vi "Get Cursor Values from Data.vi"(5 "octave spectra":T5(array[cluster]) {"band power" format="%.2f"; "nominal frequencies [Hz]" format="%.2f"}, 7 "octave info":T6[](array[typedef]) {"engineering units" items=["custom..."=0, "V"=1, "A"=21, "C"=30, "pC"=31, "s"=32, "-"=29, "Pa"=2, "N"=20, "g"=3, "m/s^2"=4, "m/s"=5, "m"=6, "mm/s"=12, "mm"=13, "micron/s"=14, "micron"=15, "in/s^2"=7, "in/s"=8, "in"=9, "mil/s"=10, "mil"=11, "rad/s^2"=16, "rad/s"=17, "rad"=18, "deg/s^2"=26, "deg/s"=27, "deg"=28, "RPM"=22, "cycle/s^2"=23, "Hz"=24, "cycle"=25, "strain"=19]; "dB reference" format="%.2e"; "weighting filter" items=["Linear", "A-weighting", "B-weighting", "C-weighting", "ITU-R 468-4", "Dolby", "CCITT", "C-message", "Wb", "Wc", "Wd", "We", "Wf", "Wh", "Wj", "Wk", "Wm", "AES17 20 kHz lowpass", "AES17 40 kHz lowpass", "AES17 20 kHz highpass", "AES17 40 kHz highpass"]}, 10 "Refnums for FP Objects":T1, 11 "Display State In":T2={"Graph Visible Items"={"Plot Legend"=FALSE, "Scale Legend"=FALSE, "Graph Palette"=FALSE, "Cursor Legend"=FALSE, "X Scrollbar"=FALSE}, "View Table"=FALSE, "Table Visible Items"={"Vertical Scrollbar"=FALSE, "Horizontal Scrollbar"=FALSE, "Row Headers"=FALSE, "Column Headers"=FALSE, "Vertical Lines"=FALSE, "Horizontal Lines"=FALSE}, "Header Font"={"Font Name"="", "Size"=0, "Bold"=FALSE, "Italic"=FALSE, "Underline"=FALSE, "Strikeout"=FALSE, "Color"=0}, "Cell Font"={"Font Name"="", "Size"=0, "Bold"=FALSE, "Italic"=FALSE, "Underline"=FALSE, "Strikeout"=FALSE, "Color"=0}, "Description and Tip..."={"Description"="", "Tip"=""}, "Moveable Splitter Position"=0, "Measurement Cursor Configuration"={"XY"={"enable XY"=FALSE, "Position (X)"=[], "Type"=enum."Absolute", "Y reference"=0.0, "color"=0}, "band"={"enable band"=FALSE, "B1"=0.0, "B2"=0.0, "Fixed bandwidth (B2-B1)"=0.0, "B1 color"=0, "B2 color"=0}, "harmonic"={"enable harmonics"=FALSE, "X reference (1X)"=0.0, "Maximum"=0, "Subset"=enum."All", "1X color"=0, "MX color"=0}, "sideband"={"enable sideband"=FALSE, "X center (C)"=0.0, "Sidebands"=0, "X spacing (s)"=0.0, "Center color"=0, "Sideband color"=0}}, "Cursors"={"List"=[], "Tags"=[]}, "X Increment"=0.0, "X Scale"={"Label Visible"=FALSE, "Label Text"="", "Mapping Mode"=0, "Format String"=""}, "Y Scale"={"Label Visible"=FALSE, "Label Text"="", "Mapping Mode"=0, "Format String"=""}, "Colors"={"background"=16777215, "major grid"=8355711, "minor grid"=12632256, "font"=0}, "desired spectrum view"={"scaling"={"linear/dB"=enum."no change", "dB reference"=0.0, "power/magnitude"=enum."no change", "view"=enum."no change"}, "spectral density"=enum."no change"}, "Plot Color Wheel"=[3381759, 32768, 982784, 4375295, 13827953, 13457919, 16757522, 4343295, 16728758, 12095254], "Plots"=[], "registered user events"=variant, "Lock 1X to Peak"=FALSE} caption="State" {"Y Scale"."Mapping Mode" items=["Linear", "Logarithmic", "dB"]; "X Scale"."Mapping Mode" items=["Linear", "Logarithmic"]}) -> (2 "value table":string[][](array[string]), 3 "Display State Out":T2={"Graph Visible Items"={"Plot Legend"=FALSE, "Scale Legend"=FALSE, "Graph Palette"=FALSE, "Cursor Legend"=FALSE, "X Scrollbar"=FALSE}, "View Table"=FALSE, "Table Visible Items"={"Vertical Scrollbar"=FALSE, "Horizontal Scrollbar"=FALSE, "Row Headers"=FALSE, "Column Headers"=FALSE, "Vertical Lines"=FALSE, "Horizontal Lines"=FALSE}, "Header Font"={"Font Name"="", "Size"=0, "Bold"=FALSE, "Italic"=FALSE, "Underline"=FALSE, "Strikeout"=FALSE, "Color"=0}, "Cell Font"={"Font Name"="", "Size"=0, "Bold"=FALSE, "Italic"=FALSE, "Underline"=FALSE, "Strikeout"=FALSE, "Color"=0}, "Description and Tip..."={"Description"="", "Tip"=""}, "Moveable Splitter Position"=0, "Measurement Cursor Configuration"={"XY"={"enable XY"=FALSE, "Position (X)"=[], "Type"=enum."Absolute", "Y reference"=0.0, "color"=0}, "band"={"enable band"=FALSE, "B1"=0.0, "B2"=0.0, "Fixed bandwidth (B2-B1)"=0.0, "B1 color"=0, "B2 color"=0}, "harmonic"={"enable harmonics"=FALSE, "X reference (1X)"=0.0, "Maximum"=0, "Subset"=enum."All", "1X color"=0, "MX color"=0}, "sideband"={"enable sideband"=FALSE, "X center (C)"=0.0, "Sidebands"=0, "X spacing (s)"=0.0, "Center color"=0, "Sideband color"=0}}, "Cursors"={"List"=[], "Tags"=[]}, "X Increment"=0.0, "X Scale"={"Label Visible"=FALSE, "Label Text"="", "Mapping Mode"=0, "Format String"=""}, "Y Scale"={"Label Visible"=FALSE, "Label Text"="", "Mapping Mode"=0, "Format String"=""}, "Colors"={"background"=16777215, "major grid"=8355711, "minor grid"=12632256, "font"=0}, "desired spectrum view"={"scaling"={"linear/dB"=enum."no change", "dB reference"=0.0, "power/magnitude"=enum."no change", "view"=enum."no change"}, "spectral density"=enum."no change"}, "Plot Color Wheel"=[3381759, 32768, 982784, 4375295, 13827953, 13457919, 16757522, 4343295, 16728758, 12095254], "Plots"=[], "registered user events"=variant, "Lock 1X to Peak"=FALSE} caption="State" {"Y Scale"."Mapping Mode" items=["Linear", "Logarithmic", "dB"]; "X Scale"."Mapping Mode" items=["Linear", "Logarithmic"]}, 4 "measurement names":string[](array[string]), 6 "channels":string[](array[string]))   [LabVIEW 2017, in "Octave with Cursors.xctl"]
doc: "This VI extracts the spectral values at the cursor positions. Based on the spectral data, Row Headers, Column Headers, and Values are written to the table."
uses:
  <vilib>/addons/_XControls/Octave with Cursors/Octave with Cursors.xctl
  <vilib>/addons/_XControls/Octave with Cursors/Controls/State.ctl
  <vilib>/Utility/miscctls.llb/LVFontTypeDef.ctl
  <vilib>/addons/_XControls/Octave with Cursors/Controls/Measurement Cursor Configuration.ctl
  <vilib>/addons/_NISVFA/_Shared subVIs/Controls/svc_Octave Info.ctl
  <vilib>/addons/_NISVFA/_Shared subVIs/Controls/svc_Octave Standard.ctl
  <vilib>/addons/_NISVFA/_Shared subVIs/Controls/svc_Weighting Filter Text Ring.ctl
  <vilib>/addons/_NISVFA/_Shared subVIs/Controls/svc_Engineering Units Text Ring.ctl
  <vilib>/addons/_XControls/Octave with Cursors/Controls/Refnums Typedef.ctl
  <vilib>/addons/Sound and Vibration/svt_Controls/subVIs/Multiplot Octave Graph.ctl
  <vilib>/Analysis/baseanly.llb/Mean (DBL).vi
  <vilib>/addons/Sound and Vibration/svt_Octave/SVT Get Octave Subset (N Ch).vi
  <vilib>/addons/Sound and Vibration/svt_Octave/SVT Get Octave Value (N Ch).vi
  <vilib>/Analysis/NI_AALBase.lvlib
  <vilib>/addons/Sound and Vibration/svt_Octave/SoundVib_Octave.lvlib
  <vilib>/addons/Sound and Vibration/svt_Octave/SoundVib_Octave_2014 standard.lvlib
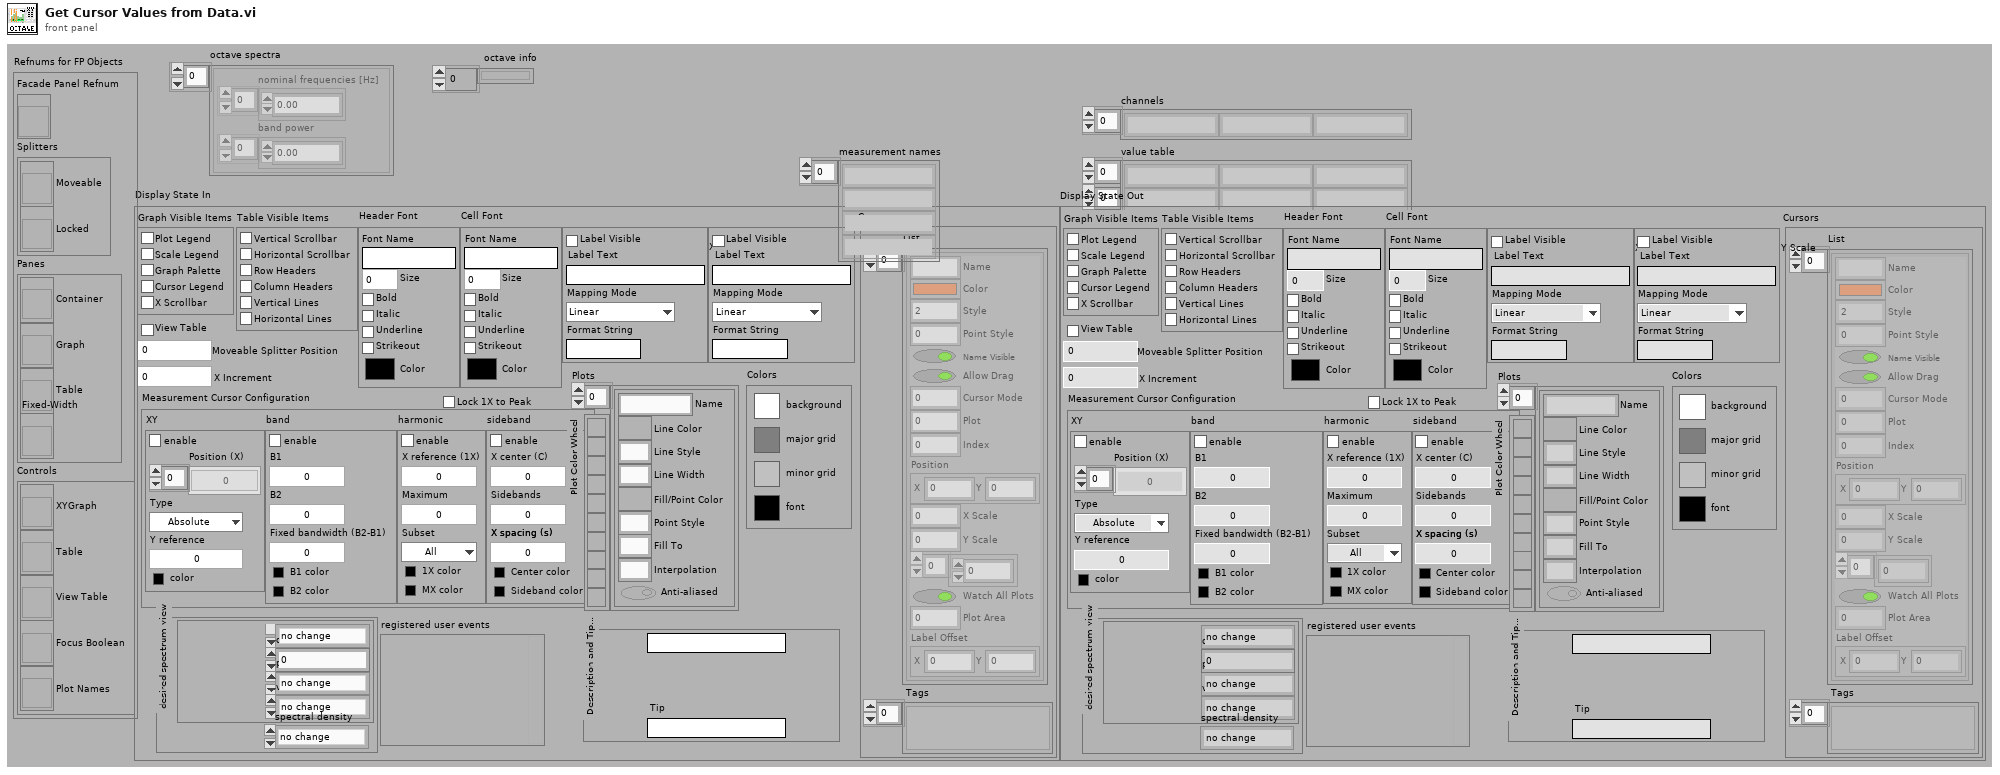
[diagram p1: front panel]
types:
  T1 = typedef "Octave with Cursors.xctl/Refnums Typedef.ctl" = cluster{"Facade Panel Refnum":refnum<vi>, "Splitters":cluster{"Moveable":refnum<vi>, "Locked":refnum<vi>}, "Panes":cluster{"Container":refnum<vi>, "Graph":refnum<vi>, "Table":refnum<vi>, "Fixed-Width":refnum<vi>}, "Controls":cluster{"XYGraph":refnum<vi>, "Table":refnum<vi>, "View Table":refnum<vi>, "Focus Boolean":refnum<vi>, "Plot Names":refnum<vi>}}
  T2 = typedef "Octave with Cursors.xctl/State.ctl" = cluster{"Graph Visible Items":cluster{"Plot Legend":bool, "Scale Legend":bool, "Graph Palette":bool, "Cursor Legend":bool, "X Scrollbar":bool}, "View Table":bool, "Table Visible Items":cluster{"Vertical Scrollbar":bool, "Horizontal Scrollbar":bool, "Row Headers":bool, "Column Headers":bool, "Vertical Lines":bool, "Horizontal Lines":bool}, "Header Font":T3, "Cell Font":T3, "Description and Tip...":cluster{"Description":string, "Tip":string}, "Moveable Splitter Position":i32, "Measurement Cursor Configuration":T4, "Cursors":cluster{"List":cluster{"Name":string, "Color":u32, "Style":i32, "Point Style":u8, "Name Visible":bool, "Allow Drag":bool, "Cursor Mode":u32, "Plot":i32, "Index":i32, "Position":cluster{"X":dbl, "Y":dbl}, "X Scale":u32, "Y Scale":u32, "Watch Plots":i32[], "Watch All Plots":bool, "Plot Area":i32, "Label Offset":cluster{"X":dbl, "Y":dbl}}[], "Tags":variant[]}, "X Increment":dbl, "X Scale":cluster{"Label Visible":bool, "Label Text":string, "Mapping Mode":u8, "Format String":string}, "Y Scale":cluster{"Label Visible":bool, "Label Text":string, "Mapping Mode":u8, "Format String":string}, "Colors":cluster{"background":u32, "major grid":u32, "minor grid":u32, "font":u32}, "desired spectrum view":cluster{"scaling":cluster{"linear/dB":enum16{"no change", "linear", "dB"}, "dB reference":dbl, "power/magnitude":enum16{"no change", "power", "magnitude"}, "view":enum16{"no change", "rms", "peak", "peak-peak"}}, "spectral density":enum16{"no change", "spectrum", "spectral density"}}, "Plot Color Wheel":u32[], "Plots":cluster{"Name":string, "Line Color":u32, "Line Style":u8, "Line Width":u8, "Fill/Point Color":u32, "Point Style":u8, "Fill To":i16, "Interpolation":u8, "Anti-aliased":bool}[], "registered user events":variant, "Lock 1X to Peak":bool}
  T3 = typedef "LVFontTypeDef.ctl" = cluster{"Font Name":string, "Size":u16, "Bold":bool, "Italic":bool, "Underline":bool, "Strikeout":bool, "Color":u32}
  T4 = typedef "Octave with Cursors.xctl/Measurement Cursor Configuration.ctl" = cluster{"XY":cluster{"enable XY":bool, "Position (X)":dbl[], "Type":enum16{"Absolute", "Relative"}, "Y reference":dbl, "color":u32}, "band":cluster{"enable band":bool, "B1":dbl, "B2":dbl, "Fixed bandwidth (B2-B1)":dbl, "B1 color":u32, "B2 color":u32}, "harmonic":cluster{"enable harmonics":bool, "X reference (1X)":dbl, "Maximum":i32, "Subset":enum16{"All", "Even", "Odd"}, "1X color":u32, "MX color":u32}, "sideband":cluster{"enable sideband":bool, "X center (C)":dbl, "Sidebands":i32, "X spacing (s)":dbl, "Center color":u32, "Sideband color":u32}}
  T5 = cluster{"nominal frequencies [Hz]":dbl[], "band power":dbl[]}[]
  T6 = typedef "svc_Octave Info.ctl" = cluster{"standard":T7, "bandwidth":enum16{"1 octave", "1/3 octave", "1/6 octave", "1/12 octave", "1/24 octave"}, "low band":i32, "high band":i32, "weighting filter":T8, "dB reference":dbl, "dB On":bool, "unit label":string, "channel name":string, "description":string, "engineering units":T9, "custom label":string, "spectrum type":enum16{"power", "magnitude"}, "spectral density":bool, "filters settled":bool}
  T7 = typedef "svc_Octave Standard.ctl" = enum16{"ANSI S1.11", "IEC 61260"}
  T8 = typedef "svc_Weighting Filter Text Ring.ctl" = u16
  T9 = typedef "svc_Engineering Units Text Ring.ctl" = u16
  T10 = enum16{"coerce to nearest", "coerce to next highest", "coerce to next lowest", "interpolate"}
  T11 = enum16{"1 octave", "1/3 octave", "1/6 octave", "1/12 octave", "1/24 octave"}
  T12 = cluster{"nominal frequencies [Hz]":dbl[], "band power":dbl[]}
  T13 = cluster{"List":cluster{"Name":string, "Color":u32, "Style":i32, "Point Style":u8, "Name Visible":bool, "Allow Drag":bool, "Cursor Mode":u32, "Plot":i32, "Index":i32, "Position":cluster{"X":dbl, "Y":dbl}, "X Scale":u32, "Y Scale":u32, "Watch Plots":i32[], "Watch All Plots":bool, "Plot Area":i32, "Label Offset":cluster{"X":dbl, "Y":dbl}}[], "Tags":variant[]}
  T14 = cluster{"Name":string, "Color":u32, "Style":i32, "Point Style":u8, "Name Visible":bool, "Allow Drag":bool, "Cursor Mode":u32, "Plot":i32, "Index":i32, "Position":cluster{"X":dbl, "Y":dbl}, "X Scale":u32, "Y Scale":u32, "Watch Plots":i32[], "Watch All Plots":bool, "Plot Area":i32, "Label Offset":cluster{"X":dbl, "Y":dbl}}[]
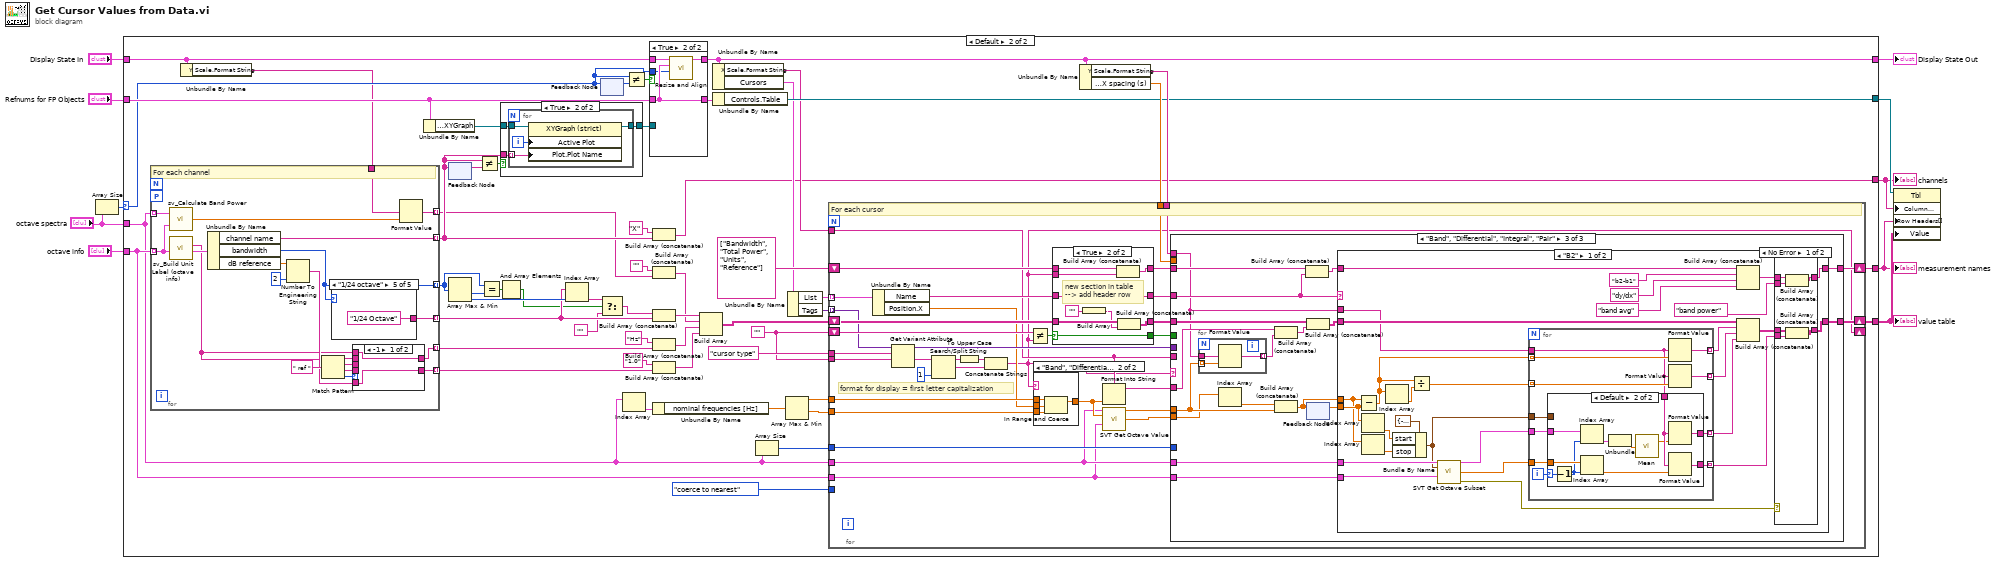
[diagram p0: block diagram]
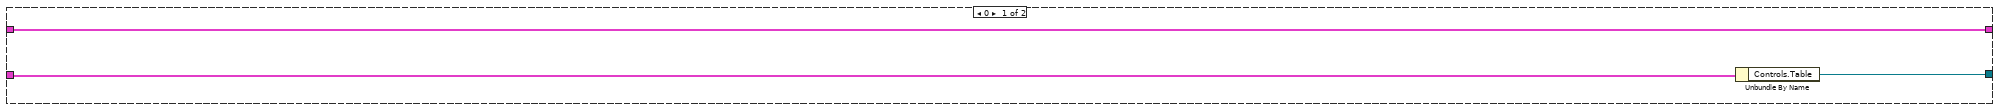
[diagram p2: hidden frame]
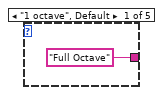
[diagram p5: hidden frame]
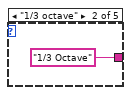
[diagram p6: hidden frame]
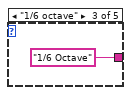
[diagram p7: hidden frame]
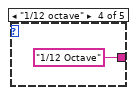
[diagram p8: hidden frame]
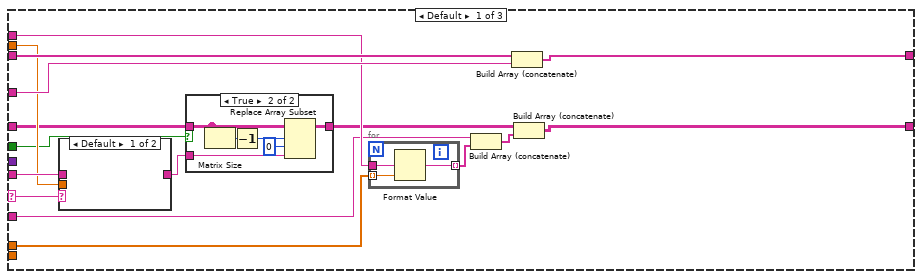
[diagram p12: hidden frame]
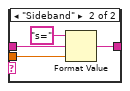
[diagram p14: hidden frame]
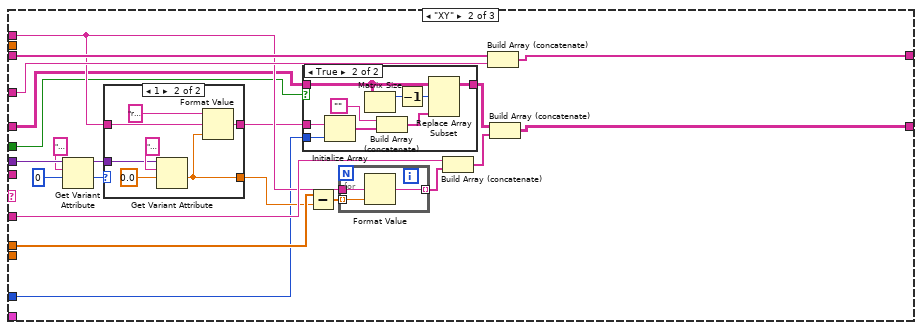
[diagram p15: hidden frame]
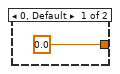
[diagram p17: hidden frame]
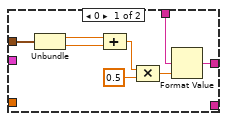
[diagram p19: hidden frame]
diagram:
  n1 = Array Size(array="octave spectra") -> (size(s)=w5:i32)
  n2 = case shown="Default" w5 {
    selector: w5 -> [_ w33]
    tunnel: "octave info" -> [_ w67]
    tunnel: [_ w60] -> w2
    tunnel: [_ w59] -> w1
    tunnel: [_ w21] -> w3
    tunnel: [w13 w38] -> w9
    tunnel: "octave spectra" -> [_ w20]
    tunnel: "Display State In" -> [w13 w17]
    tunnel: "Refnums for FP Objects" -> [w12 w37]
    tunnel: [w11 w40] -> w4
    frame 0 {
      n3 = Unbundle By Name(w12) -> ("Controls.Table"=w11:refnum<vi>)
    }
    frame Default {
      w58 = "" ("String")
      n4 = Unbundle By Name(w17) -> ("Y Scale.Format String"=w16:string)
      n5 = for {
        tunnel: w67 -> [w86] mode=indexing
        tunnel: [w92] -> w27 mode=indexing
        tunnel: [w95] -> w65 mode=indexing
        tunnel: [w88] -> w46 mode=indexing
        tunnel: [w94] -> w56 mode=indexing
        tunnel: [w89] -> w42 mode=indexing
        workers-P: _ -> [_]
        tunnel: w20 -> [w87] mode=indexing
        tunnel: w16 -> [w84]
        tunnel: [w83] -> w15 mode=indexing
        # "For each channel"
        n6 = Format Value() -> ()  [unwired: 3 in, 1 out]
        n7 = call <vilib>:"sv_Calculate Band Power.vi"("octave info"=w86, "octave spectrum"=w87) -> ("total band power"=w85:dbl)
        n8 = call <vilib>:"sv_Build Unit Label (octave info).vi"("octave info"=w86) -> ("octave info out"=w91:T6, "unit label"=w90:string)  [unwired: 8 in, 1 out]
        n9 = Unbundle By Name(w91) -> ("channel name"=w92:string, "bandwidth"=w89:T11, "dB reference"=w101:dbl)
        n10 = Number To Engineering String(2:i16 2 ("precision (6)"), 4:w101) -> (0:w93:string)  [unwired: 2 in]
        n11 = Match Pattern(string=w90, regular expression=" ref ") -> (before substring=w98:string, match substring=w97:string, after substring=w96:string, offset past match=w99:i32)  [unwired: 1 in]
        n12 = case shown="\"1/24 octave\"" w89 {
          tunnel: ["Full Octave" ("String") "1/3 Octave" ("String") "1/6 Octave" ("String") "1/12 Octave" ("String") "1/24 Octave" ("String")] -> w88
          frame "1 octave", Default {
          }
          frame "1/3 octave" {
          }
          frame "1/6 octave" {
          }
          frame "1/12 octave" {
          }
          frame "1/24 octave" {
          }
        }
        n13 = case shown="-1" w99 {
          tunnel: w98 -> [_ w111]
          tunnel: w97 -> [_ _]
          tunnel: w96 -> [_ w110]
          tunnel: [w109 w111] -> w95
          tunnel: w90 -> [w109 _]
          tunnel: [w108 w110] -> w94
          tunnel: w93 -> [w108 _]
          frame -1 {
          }
          frame Default {
          }
        }
        n14 = Format Value(format string=w84, value (0)=w85) -> (output string=w83:string)  [unwired: 1 in]
      }
      n15 = Unbundle By Name(w37) -> ("Controls.XYGraph"=w41:refnum<vi>)
      n16 = feedback #1() -> (w29:string[])  [unwired: 1 in]
      n17 = feedback-in #1(w27) -> ()
      n18 = Array Max & Min(array=w42) -> (min value=w50:T11, min index (indices)=w48:i32)  [unwired: 2 out]
      n19 = Not Equal?(x=w27, y=w29) -> (x != y?=w28:bool)
      n20 = Equal?(x=w42, y=w50) -> (x = y?=w49:bool[])
      n21 = And Array Elements(Boolean array=w49) -> (logical AND=w45:bool)
      n22 = case shown="True" w28 {
        tunnel: w41 -> [w69 w72]
        tunnel: [w69 w71] -> w34
        tunnel: w27 -> [_ w70]
        frame False {
        }
        frame True {
          n23 = for {
            tunnel: w72 -> [w76]
            tunnel: w70 -> [w74] mode=indexing
            tunnel: [w73] -> w71
            i -> [w75]
            n24 = property class="XYGraph (strict)"(reference=w76, "Active Plot"=w75, "Plot.Plot Name"=w74) -> (reference out=w73:refnum<vi>)  [unwired: 1 in, 1 out]
          }
        }
      }
      n25 = Index Array(array=w46, index=w48) -> (element=w47:string)
      n26 = feedback #2() -> (w52:i32)  [unwired: 1 in]
      n27 = feedback-in #2(w33) -> ()
      n28 = Select(t=w47, s=w45, f="" ("String")) -> (s? t:f=w44:string)
      n29 = Index Array(array=w20) -> (element=w25:T12)  [unwired: 1 in]
      n30 = Not Equal?(x=w33, y=w52) -> (x != y?=w35:bool)
      n31 = case shown="True" w35 {
        tunnel: w17 -> [w78 w82]
        tunnel: [w78 w81] -> w38
        tunnel: w37 -> [w77 w80]
        tunnel: [w77 w80] -> w36
        tunnel: w33 -> [_ w79]
        tunnel: w34 -> [_ _]
        frame False {
        }
        frame True {
          n32 = call <vilib>:"Resize and Align.vi"("number of channels"=w79, "Refnums for Resizing and Alignment"=w80, "State in"=w82) -> ("State out"=w81:T2)  [unwired: 7 in, 1 out]
        }
      }
      n33 = Build Array (concatenate)("X" ("String"), w27) -> (w21:string[])
      n34 = Build Array (concatenate)("" ("String"), w15) -> (w14:string[])
      n35 = Build Array (concatenate)(w44, w46) -> (w61:string[])
      n36 = Build Array (concatenate)("Hz" ("String"), w65) -> (w64:string[])
      n37 = Build Array (concatenate)("1.0" ("String"), w56) -> (w57:string[])
      n38 = Unbundle By Name(w25) -> ("nominal frequencies [Hz]"=w24:dbl[])
      n39 = Build Array(w61, w14, w64, w57) -> (w19:string[][])
      n40 = Unbundle By Name(w38) -> ("X Scale.Format String"=w39:string, "Cursors"=w32:T13)
      n41 = Unbundle By Name(w36) -> ("Controls.Table"=w40:refnum<vi>)
      n42 = Array Size(array=w20) -> (size(s)=w54:i32)
      n43 = Array Max & Min(array=w24) -> (max value=w23:dbl, min value=w22:dbl)  [unwired: 2 out]
      n44 = Unbundle By Name(w32) -> ("List"=w31:T14, "Tags"=w30:variant[])
      n45 = Unbundle By Name(w38) -> ("Y Scale.Format String"=w55:string, "Measurement Cursor Configuration.sideband.X spacing (s)"=w53:dbl)
      n46 = for {
        tunnel: w20 -> [w113]
        tunnel: w67 -> [w112]
        tunnel: T10."coerce to nearest" ("frequency coercion") -> [_]
        shift-right: [w145] -> w59
        shift-left: string[] ["Bandwidth", "Total Power", "Units", "Reference"] ("Array") -> [w137]
        shift-right: [w144] -> w60
        shift-left: w19 -> [w138]
        tunnel: "cursor type" -> [w143]
        shift-right: [w114] -> _
        shift-left: w58 -> [w142]
        tunnel: w58 -> [w141]
        tunnel: w39 -> [w115]
        tunnel: w55 -> [w127]
        tunnel: w54 -> [w125]
        tunnel: w53 -> [w124]
        tunnel: w22 -> [w121]
        tunnel: w23 -> [w120]
        tunnel: w31 -> [w119] mode=indexing
        tunnel: w30 -> [w116] mode=indexing
        # "format for display = first letter capitalization"
        # "For each cursor"
        n47 = Unbundle By Name(w119) -> ("Name"=w118:string, "Position.X"=w117:dbl)
        n48 = Get Variant Attribute(Variant=w116, name=w143, default value (empty Variant)=w141) -> (duplicate Variant=w129:variant, value=w130:string)  [unwired: 1 in, 2 out]
        n49 = Search/Split String(string=w130, offset (0)=1) -> (substring before match=w133:string, match + rest of string=w131:string)  [unwired: 1 in, 1 out]
        n50 = To Upper Case(1:w133) -> (0:w132:string)
        n51 = Concatenate Strings(w132, w131) -> (w114:string)
        n52 = Not Equal?(x=w142, y=w114) -> (x != y?=w140:bool)
        n53 = case shown="\"Band\", \"Differential\", \"Integral\", \"Pair\"" w114 {
          tunnel: w117 -> [w147 w151]
          tunnel: [w147 w150] -> w122
          tunnel: w121 -> [_ w149]
          tunnel: w120 -> [_ w148]
          frame Default {
          }
          frame "Band", "Differential", "Integral", "Pair" {
            n54 = In Range and Coerce(upper limit=w148, x=w151, lower limit=w149) -> (coerced(x)=w150:dbl)  [unwired: 1 out]
          }
        }
        n55 = case shown="True" w140 {
          selector: w140 -> [w152 w156]
          tunnel: [w155 w164] -> w139
          tunnel: w118 -> [w155 w164]
          tunnel: w138 -> [w153 w159]
          tunnel: w137 -> [w154 w162]
          tunnel: [w154 w163] -> w136
          tunnel: [w153 w160] -> w135
          tunnel: w114 -> [_ w161]
          tunnel: [w152 w156] -> w126
          frame False {
          }
          frame True {
            # "new section in table\n--> add header row"
            n56 = Build Array("") -> (w157:string[])
            n57 = Build Array (concatenate)(w162, w161) -> (w163:string[])
            n58 = Build Array (concatenate)(w159, w157) -> (w160:string[][])
          }
        }
        n59 = Format Into String(format string=w115, w122) -> (resulting string=w128:string)  [unwired: 2 in, 1 out]
        n60 = call-poly <vilib>:"SVT Get Octave Value.vi"("octave spectra"=w113, "frequency [Hz]"=w122, "octave info"=w112) -> ("band power values"=w146:dbl[], "actual nominal frequencies [Hz]"=w123:dbl[])  [unwired: 9 in, 2 out]
        n61 = case shown="\"Band\", \"Differential\", \"Integral\", \"Pair\"" w114 {
          selector: w114 -> [w172 _ _]
          tunnel: w146 -> [w174 w211 w249]
          tunnel: w136 -> [w180 w215 w254]
          tunnel: w139 -> [w179 w214 w248]
          tunnel: [w178 w213 w247] -> w145
          tunnel: w135 -> [w168 w198 w253]
          tunnel: [w177 w212 w244] -> w144
          tunnel: w129 -> [_ w210 _]
          tunnel: w128 -> [w171 w205 w251]
          tunnel: w127 -> [w175 w200 w239]
          tunnel: w126 -> [w166 w199 _]
          tunnel: w125 -> [_ w195 _]
          tunnel: w115 -> [w170 _ _]
          tunnel: w124 -> [w169 _ _]
          tunnel: w123 -> [_ _ w243]
          tunnel: w113 -> [_ _ w238]
          tunnel: w112 -> [_ _ w237]
          frame Default {
            n62 = case shown="Default" w172 {
              tunnel: w170 -> [_ w190]
              tunnel: w169 -> [_ w189]
              tunnel: [_ w188] -> w165
              frame Default {
              }
              frame "Sideband" {
                n63 = Format Value(string ("")="s=", format string=w190, value (0)=w189) -> (output string=w188:string)
              }
            }
            n64 = case shown="True" w166 {
              tunnel: w168 -> [w181 w185]
              tunnel: [w181 w187] -> w167
              tunnel: w165 -> [_ w183]
              frame False {
              }
              frame True {
                n65 = Matrix Size(0:w185) -> (1:w186:i32)  [unwired: 1 out]
                n66 = Decrement(x=w186) -> (x-1=w184:i32)
                n67 = Replace Array Subset(array=w185, new element=w183, index (row)=w184, index (col)=0 ("disabled index (col)")) -> (w187:string[][])
              }
            }
            n68 = for {
              tunnel: w174 -> [w194] mode=indexing
              tunnel: [w193] -> w176 mode=indexing
              tunnel: w175 -> [w192]
              n69 = Format Value(format string=w192, value (0)=w194) -> (output string=w193:string)  [unwired: 1 in]
            }
            n70 = Build Array (concatenate)(w171, w176) -> (w173:string[])
            n71 = Build Array (concatenate)(w180, w179) -> (w178:string[])
            n72 = Build Array (concatenate)(w167, w173) -> (w177:string[][])
          }
          frame "XY" {
            n73 = Get Variant Attribute(Variant=w210, name="xy type", default value (empty Variant)=u16 0 ("precision (6)")) -> (duplicate Variant=w209:variant, value=w206:u16)  [unwired: 1 in, 2 out]
            n74 = case shown="1" w206 {
              tunnel: [0.0 ("element") w231] -> w203
              tunnel: w209 -> [_ w234]
              tunnel: w200 -> [_ w232]
              tunnel: [_ w230] -> w196
              frame 0, Default {
              }
              frame 1 {
                n75 = Get Variant Attribute(Variant=w234, name="y reference", default value (empty Variant)=0.0 ("element")) -> (value=w231:dbl)  [unwired: 1 in, 3 out]
                n76 = Format Value(string ("")="ref=", format string=w232, value (0)=w231) -> (output string=w230:string)
              }
            }
            n77 = case shown="True" w199 {
              tunnel: w198 -> [w216 w221]
              tunnel: [w216 w225] -> w197
              tunnel: w196 -> [_ w224]
              tunnel: w195 -> [_ w223]
              frame False {
              }
              frame True {
                n78 = Initialize Array(w224, w223) -> (w219:string[])
                n79 = Matrix Size(0:w221) -> (1:w222:i32)  [unwired: 1 out]
                n80 = Build Array (concatenate)("", w219) -> (w217:string[])
                n81 = Decrement(x=w222) -> (x-1=w220:i32)
                n82 = Replace Array Subset(array=w221, new element=w217, index (row)=w220) -> (w225:string[][])  [unwired: 1 in]
              }
            }
            n83 = Subtract(x=w211, y=w203) -> (x-y=w202:dbl[])
            n84 = for {
              tunnel: w202 -> [w228] mode=indexing
              tunnel: [w227] -> w201 mode=indexing
              tunnel: w200 -> [w226]
              n85 = Format Value(format string=w226, value (0)=w228) -> (output string=w227:string)  [unwired: 1 in]
            }
            n86 = Build Array (concatenate)(w205, w201) -> (w204:string[])
            n87 = Build Array (concatenate)(w215, w214) -> (w213:string[])
            n88 = Build Array (concatenate)(w197, w204) -> (w212:string[][])
          }
          frame "Band", "Differential", "Integral", "Pair" {
            n89 = for {
              tunnel: w249 -> [w326] mode=indexing
              tunnel: [w325] -> w252 mode=indexing
              tunnel: w239 -> [w324]
              n90 = Format Value(format string=w324, value (0)=w326) -> (output string=w325:string)  [unwired: 1 in]
            }
            n91 = Index Array(array=w243) -> (element=w242:dbl)  [unwired: 1 in]
            n92 = Build Array (concatenate)(w251, w252) -> (w250:string[])
            n93 = Build Array (concatenate)(w242, w249) -> (w241:dbl[])
            n94 = Build Array (concatenate)(w254, w248) -> (w246:string[])
            n95 = Build Array (concatenate)(w253, w250) -> (w245:string[][])
            n96 = feedback-in #3(w241) -> ()
            n97 = feedback #3() -> (w240:dbl[])  [unwired: 1 in]
            n98 = case shown="\"B2\"" w248 {
              tunnel: [w264 w323] -> w247
              tunnel: w246 -> [w283 w323]
              tunnel: w245 -> [w281 w322]
              tunnel: [w261 w322] -> w244
              tunnel: w241 -> [w271 _]
              tunnel: w240 -> [w273 _]
              tunnel: w239 -> [w279 _]
              tunnel: w238 -> [w258 _]
              tunnel: w237 -> [w259 _]
              frame "B2" {
                n99 = Subtract(x=w271, y=w273) -> (x-y=w277:dbl[])
                n100 = Index Array(array=w273) -> (element=w272:dbl)  [unwired: 1 in]
                n101 = Index Array(array=w271) -> (element=w270:dbl)  [unwired: 1 in]
                n102 = Index Array(array=w277) -> (element=w278:dbl)  [unwired: 1 in]
                n103 = Bundle By Name(cluster=cluster{"start":dbl, "stop":dbl} {"start"=-1.0, "stop"=-1.0} ("range"), "start"=w272, "stop"=w270) -> (w255:cluster{"start":dbl, "stop":dbl})
                n104 = Divide(x=w277, y=w278) -> (x/y=w276:dbl[])
                n105 = call-poly <vilib>:"SVT Get Octave Subset.vi"("octave spectra"=w258, "frequency range [Hz]"=w255, "octave info in"=w259) -> ("octave spectra subsets"=w269:T5, "total band powers"=w256:dbl[], "error out"=w257:errorcluster)  [unwired: 8 in, 2 out]
                n106 = for {
                  tunnel: w277 -> [w302] mode=indexing
                  tunnel: [w301] -> w280 mode=indexing
                  tunnel: w279 -> [w295]
                  tunnel: w276 -> [w300] mode=indexing
                  tunnel: [w299] -> w275 mode=indexing
                  tunnel: w269 -> [w297]
                  tunnel: w256 -> [w296]
                  tunnel: [w294] -> w260 mode=indexing
                  tunnel: [w293] -> w268 mode=indexing
                  tunnel: w255 -> [w292]
                  i -> [w298]
                  n107 = case shown="Default" w298 {
                    selector: w298 -> [_ w321]
                    tunnel: w297 -> [_ w320]
                    tunnel: w296 -> [_ w319]
                    tunnel: w295 -> [w307 w318]
                    tunnel: [_ w316] -> w294
                    tunnel: [w306 w315] -> w293
                    tunnel: w292 -> [w305 _]
                    frame 0 {
                      n108 = Unbundle(w305) -> ("start"=w304:dbl, "stop"=w303:dbl)
                      n109 = Compound Arithmetic op=ADD(w304, w303) -> (w310:dbl)
                      n110 = Compound Arithmetic op=MULTIPLY(w310, 0.5 ("value")) -> (w308:dbl)
                      n111 = Format Value(format string=w307, value (0)=w308) -> (output string=w306:string)  [unwired: 1 in]
                    }
                    frame Default {
                      n112 = Decrement(x=w321) -> (x-1=w312:i32)
                      n113 = Index Array(array=w320, index=w312) -> (element=w314:T12)
                      n114 = Index Array(array=w319, index=w312) -> (element=w317:dbl)
                      n115 = Unbundle(w314) -> ("band power"=w311:dbl[])  [unwired: 1 out]
                      n116 = call-poly <vilib>:"Mean.vi"("X"=w311) -> ("mean"=w313:dbl)  [unwired: 1 out]
                      n117 = Format Value(format string=w318, value (0)=w313) -> (output string=w315:string)  [unwired: 1 in]
                      n118 = Format Value(format string=w318, value (0)=w317) -> (output string=w316:string)  [unwired: 1 in]
                    }
                  }
                  n119 = Format Value(format string=w295, value (0)=w302) -> (output string=w301:string)  [unwired: 1 in]
                  n120 = Format Value(format string=w295, value (0)=w300) -> (output string=w299:string)  [unwired: 1 in]
                }
                n121 = Build Array (concatenate)(w283, "b2-b1", "dy/dx", "band avg") -> (w265:string[])
                n122 = Build Array (concatenate)(w281, w280, w275, w268) -> (w262:string[][])
                n123 = case shown="No Error" w257 {
                  tunnel: w265 -> [w289 w291]
                  tunnel: [w288 w291] -> w264
                  tunnel: "band power" -> [w287 _]
                  tunnel: w262 -> [w286 w290]
                  tunnel: [w285 w290] -> w261
                  tunnel: w260 -> [w284 _]
                  frame No Error {
                    n124 = Build Array (concatenate)(w289, w287) -> (w288:string[])
                    n125 = Build Array (concatenate)(w286, w284) -> (w285:string[][])
                  }
                  frame Error {
                  }
                }
              }
              frame "B1", Default {
              }
            }
          }
        }
      }
    }
  }
  "channels" <- w3
  "measurement names" <- w1
  "value table" <- w2
  "Display State Out" <- w9
  n126 = property class="Tbl"(reference=w4, "Column Headers[]"=w3, "Row Headers[]"=w1, "Value"=w2) -> ()  [unwired: 1 in, 2 out]
